vi "Log Robot.vi"   [LabVIEW 2014]
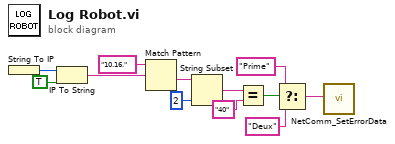
[diagram p0: block diagram]
diagram:
  n1 = String To IP() -> (0:w1:u32)  [unwired: 1 in]
  n2 = IP To String(1:TRUE ("dot notation? (F)"), 2:w1) -> (0:w2:string)
  n3 = Match Pattern(string="10.16.", regular expression=w2) -> (after substring=w4:string)  [unwired: 1 in, 3 out]
  n4 = String Subset(string=w4, length (rest)=2 ("length (rest)")) -> (substring=w6:string)  [unwired: 1 in]
  n5 = Equal?(x=w6, y="40") -> (x = y?=w8:bool)
  n6 = Select(t="Prime" ("y"), s=w8, f="Deux" ("y")) -> (s? t:f=w11:string)
  n7 = call <vilib>:"NetComm_SetErrorData.vi"("Error Data"=w11) -> ()  [unwired: 3 in, 8 out]
